vi "ChangeFlagDB.vi"(11 "ChangeFlagName":string) -> (3 "ChangeFlagQ":refnum<queue>)   [LabVIEW 2017, in "Communicable State Machine.lvlib"]
uses:
  Communicable State Machine.lvlib
  _Shared/CSM Shared.lvlib
panel:
  out "Array 2":refnum<queue>[](array[refnum])
  out "Array":string[](array[string])
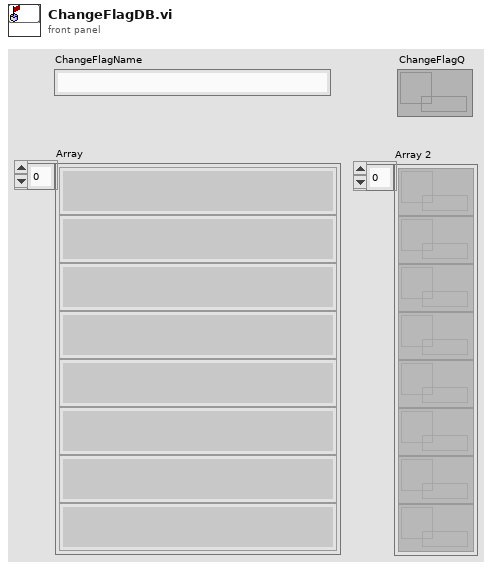
[diagram p1: front panel]
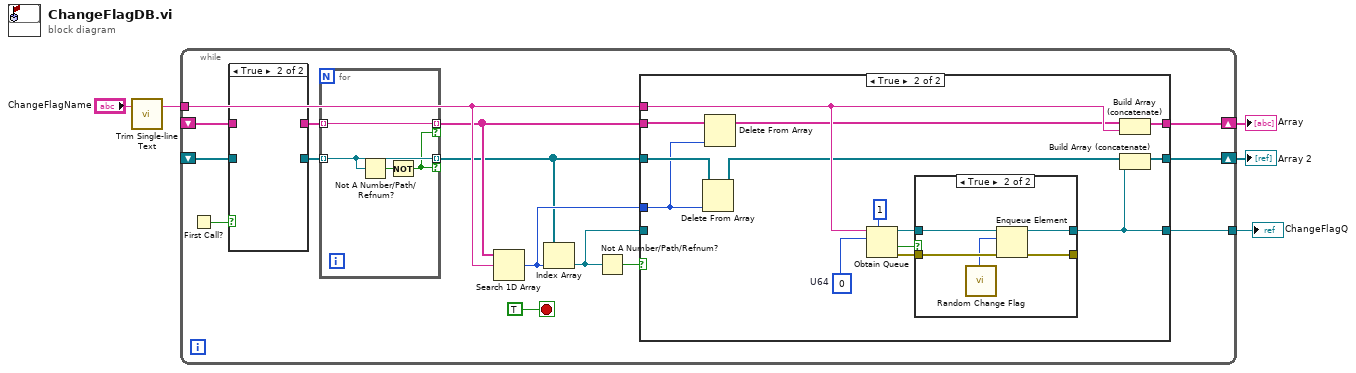
[diagram p0: block diagram]
diagram:
  n1 = call "Trim Single-line Text.vi"("single-line text"="ChangeFlagName") -> ("trimed text"=w1:string)  [unwired: 2 in]
  n2 = while {
    tunnel: w1 -> [w17]
    shift-right: [w19] -> w2
    shift-left: _ -> [w7]
    shift-right: [w18] -> w3
    shift-left: _ -> [w8]
    tunnel: [w15] -> w4
    stop <- TRUE stop-if-true
    n3 = First Call?() -> (First Call?: T/F=w10:bool)
    n4 = case shown="True" w10 {
      tunnel: [w22 _] -> w9
      tunnel: w8 -> [w22 _]
      tunnel: w7 -> [w21 _]
      tunnel: [w21 _] -> w6
      frame False {
      }
      frame True {
      }
    }
    n5 = for {
      tunnel: [w26] -> w12 mode=indexing if=w23
      tunnel: w9 -> [w26] mode=indexing
      tunnel: [w25] -> w11 mode=indexing if=w23
      tunnel: w6 -> [w25] mode=indexing
      n6 = Not A Number/Path/Refnum?(number/path/refnum=w25) -> (NaN/Path/Refnum?=w24:bool)
      n7 = Not(x=w24) -> (.not. x?=w23:bool)
    }
    n8 = Search 1D Array(1D array=w12, element=w17) -> (index of element=w13:i32)  [unwired: 1 in]
    n9 = Index Array(array=w11, index=w13) -> (element=w14:refnum<queue>)
    n10 = Not A Number/Path/Refnum?(number/path/refnum=w14) -> (NaN/Path/Refnum?=w16:bool)
    n11 = case shown="True" w16 {
      tunnel: w17 -> [_ w36]
      tunnel: [w29 w38] -> w19
      tunnel: w11 -> [w29 w34]
      tunnel: w12 -> [w28 w32]
      tunnel: [w28 w37] -> w18
      tunnel: [w27 w35] -> w15
      tunnel: w14 -> [w27 _]
      tunnel: w13 -> [_ w30]
      frame False {
      }
      frame True {
        w43 = u64 0  # U64
        n12 = Delete From Array(array=w34, index=w30) -> (array with subset deleted=w33:refnum<queue>[])  [unwired: 1 in, 1 out]
        n13 = Delete From Array(array=w32, index=w30) -> (array with subset deleted=w31:string[])  [unwired: 1 in, 1 out]
        n14 = Obtain Queue(max queue size (-1, unlimited)=1, name (unnamed)=w36, element data type=w43) -> (queue out=w41:refnum<queue>, created new?=w39:bool, error out=w40:errorcluster)  [unwired: 2 in]
        n15 = case shown="True" w39 {
          tunnel: w41 -> [w45 w50]
          tunnel: [w45 w49] -> w35
          tunnel: w40 -> [w44 w48]
          tunnel: [w44 w46] -> _
          frame False {
          }
          frame True {
            n16 = call "Random Change Flag.vi"() -> ("Random Change Flag"=w47:u64)  [unwired: 2 in]
            n17 = Enqueue Element(queue=w50, element=w47, error in (no error)=w48) -> (queue out=w49:refnum<queue>, error out=w46:errorcluster)  [unwired: 1 in, 1 out]
          }
        }
        n18 = Build Array (concatenate)(w31, w36) -> (w37:string[])
        n19 = Build Array (concatenate)(w33, w35) -> (w38:refnum<queue>[])
      }
    }
  }
  "ChangeFlagQ" <- w4
  "Array" <- w3
  "Array 2" <- w2
